vi "HEWH Hyperterminal.vi"(11 "Water Heater GEA2 Data In":T1 {"Hyperterminal Data"."CRC" format="%x"; "Hyperterminal Data"."Length" format="%x"; "Hyperterminal Data"."Command" format="%x"; "Hyperterminal Data"."Destination" format="%x"; "Hyperterminal Data"."Source" format="%x"}) -> (2 "Hyperterminal Data":string[][](array[string]), 3 "Water Heater GEA2 Data Out":T1 {"Hyperterminal Data"."CRC" format="%x"; "Hyperterminal Data"."Length" format="%x"; "Hyperterminal Data"."Command" format="%x"; "Hyperterminal Data"."Destination" format="%x"; "Hyperterminal Data"."Source" format="%x"})   [LabVIEW 2016]
uses:
  Utility/GEA2 Commands/HEWH/Type Definitions/GEA2 Commands WaterHeater GEA2 Data.ctl
  Utility/GEA2 Commands/HEWH/Type Definitions/GEA2 Commands Button Status.ctl
  Utility/GEA2 Commands/HEWH/Type Definitions/GEA2 Commands Status Query.ctl
  Utility/GEA2 Commands/HEWH/Type Definitions/GEA2 Commands Service Error Codes.ctl
  Utility/LabVIEW GEA2 Toolkit v1.0.0.0/library/GEA2_Toolkit.lvlib
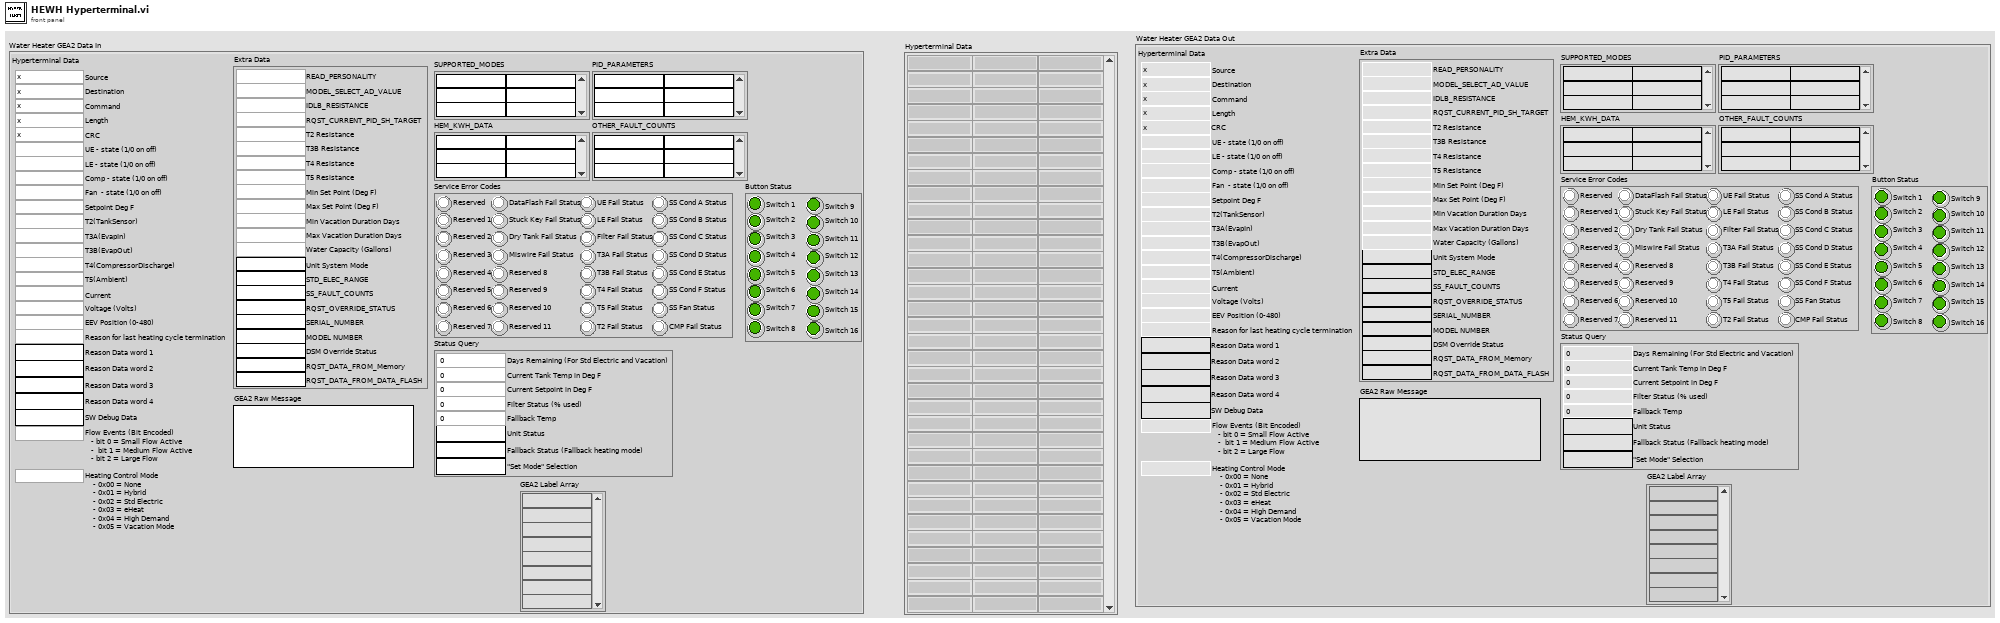
[diagram p1: front panel]
types:
  T1 = typedef "GEA2 Commands WaterHeater GEA2 Data.ctl" = cluster{"GEA2 Label Array":string[], "PID_PARAMETERS":string[][], "SUPPORTED_MODES":string[][], "Button Status":T2, "Status Query":T3, "Service Error Codes":T4, "HEM_KWH_DATA":string[][], "OTHER_FAULT_COUNTS":string[][], "GEA2 Raw Message":string, "Hyperterminal Data":cluster{"Source":u8, "Destination":u8, "Command":u8, "Length":u8, "CRC":u16, "UE - state (1/0 on off)":u8, "LE - state (1/0 on off)":u8, "Comp - state (1/0 on off)":u8, "Fan  - state (1/0 on off)":u8, "Setpoint Deg F":i32, "T2(TankSensor)":dbl, "T3A(EvapIn)":dbl, "T3B(EvapOut)":dbl, "T4(CompressorDischarge)":dbl, "T5(Ambient)":dbl, "Current":dbl, "Voltage (Volts)":u16, "EEV Position (0-480)":u16, "Reason for last heating cycle termination":u16, "Reason Data word 1":string, "Reason Data word 2":string, "Reason Data word 3":string, "Reason Data word 4":string, "SW Debug Data":string, "Flow Events (Bit Encoded)":u16, "Heating Control Mode":u16}, "Extra Data":cluster{"Water Capacity (Gallons)":u32, "Max Vacation Duration Days":u32, "Min Vacation Duration Days":u32, "Max Set Point (Deg F)":u32, "Min Set Point (Deg F)":u32, "T5 Resistance":u32, "T4 Resistance":u32, "T3B Resistance":u32, "T2 Resistance":u32, "STD_ELEC_RANGE":string, "SS_FAULT_COUNTS":string, "SERIAL_NUMBER":string, "READ_PERSONALITY":u8, "RQST_OVERRIDE_STATUS":string, "MODEL_SELECT_AD_VALUE":u32, "MODEL NUMBER":string, "IDLB_RESISTANCE":u32, "DSM Override Status":string, "RQST_DATA_FROM_Memory":string, "RQST_DATA_FROM_DATA_FLASH":string, "RQST_CURRENT_PID_SH_TARGET":u16, "Unit System Mode":string}}
  T2 = typedef "GEA2 Commands Button Status.ctl" = cluster{"Switch 1":bool, "Switch 2":bool, "Switch 3":bool, "Switch 4":bool, "Switch 5":bool, "Switch 6":bool, "Switch 7":bool, "Switch 8":bool, "Switch 9":bool, "Switch 10":bool, "Switch 11":bool, "Switch 12":bool, "Switch 13":bool, "Switch 14":bool, "Switch 15":bool, "Switch 16":bool}
  T3 = typedef "GEA2 Commands Status Query.ctl" = cluster{"Days Remaining (For Std Electric and Vacation)":u8, "Unit Status":string, "Current Tank Temp in Deg F":u8, "Current Setpoint in Deg F":u8, "Filter Status (% used)":u8, "Fallback Status (Fallback heating mode)":string, "Fallback Temp":u8, "\"Set Mode\" Selection":string}
  T4 = typedef "GEA2 Commands Service Error Codes.ctl" = cluster{"Reserved":bool, "Reserved 1":bool, "Reserved 2":bool, "Reserved 3":bool, "Reserved 4":bool, "Reserved 5":bool, "Reserved 6":bool, "Reserved 7":bool, "DataFlash Fail Status":bool, "Stuck Key Fail Status":bool, "Dry Tank Fail Status":bool, "Miswire Fail Status":bool, "Reserved 8":bool, "Reserved 9":bool, "Reserved 10":bool, "Reserved 11":bool, "UE Fail Status":bool, "LE Fail Status":bool, "Filter Fail Status":bool, "T3A Fail Status":bool, "T3B Fail Status":bool, "T4 Fail Status":bool, "T5 Fail Status":bool, "T2 Fail Status":bool, "SS Cond A Status":bool, "SS Cond B Status":bool, "SS Cond C Status":bool, "SS Cond D Status":bool, "SS Cond E Status":bool, "SS Cond F Status":bool, "SS Fan Status":bool, "CMP Fail Status":bool}
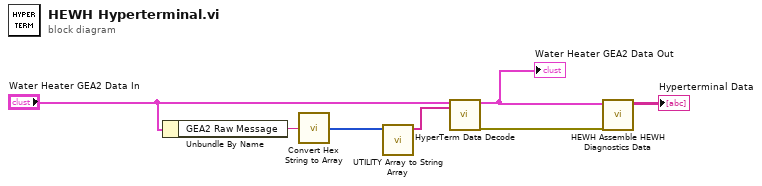
[diagram p0: block diagram]
diagram:
  n1 = Unbundle By Name("Water Heater GEA2 Data In") -> ("GEA2 Raw Message"=w6:string)
  n2 = call "Convert Hex String to Array.vi"("Hex String In"=w6) -> ("Hex Array Out"=w3:u8[])  [unwired: 14 in]
  n3 = call "UTILITY Array to String Array.vi"("Hex Array Out"=w3) -> ("Array"=w5:string[])  [unwired: 9 in, 1 out]
  n4 = call "HyperTerm Data Decode.vi"("Water Heater GEA2 Data in"="Water Heater GEA2 Data In", "Hex Array Out"=w5) -> ("Water Heater GEA2 Data out"=w4:T1, "Error Out"=w1:errorcluster)  [unwired: 16 in]
  "Water Heater GEA2 Data Out" <- w4
  n5 = call "HEWH Assemble HEWH Diagnostics Data.vi"("Error In"=w1, "Water Heater GEA2 Data in"=w4) -> ("Hyperterminal Data"=→"Hyperterminal Data":string[][])  [unwired: 8 in, 1 out]
